vi "Configure Bus Monitor.vi"(6 "Starting Address Offset":u16 format="%04x", 7 "Virtual Memory Unit in":refnum<class "Virtual Memory Unit.lvclass">, 8 "error in (no error)":errorcluster, 11 "Bus Monitor in":refnum<class "Bus Monitor.lvclass">) -> (0 "error out":errorcluster, 3 "Bus Monitor out":refnum<class "Bus Monitor.lvclass">, 5 "Virtual Memory Unit out":refnum<class "Virtual Memory Unit.lvclass">)   [LabVIEW 2020, in "BCI-1553 API.lvlib" / "Bus Monitor.lvclass"]
doc: "Configures the Bus Monitor. The Bus Monitor defaults to every command being filtered out, with new commands being filtered in based on the filters contained in this Bus Monitor at this time. The Bus Monitor will make space for 250 commands (1000-2000 addresses) and 750 data fields (26250 addresses)."
uses:
  Bus Monitor.lvclass
  Dependencies/Virtual Memory Unit/Virtual Memory Unit.lvclass
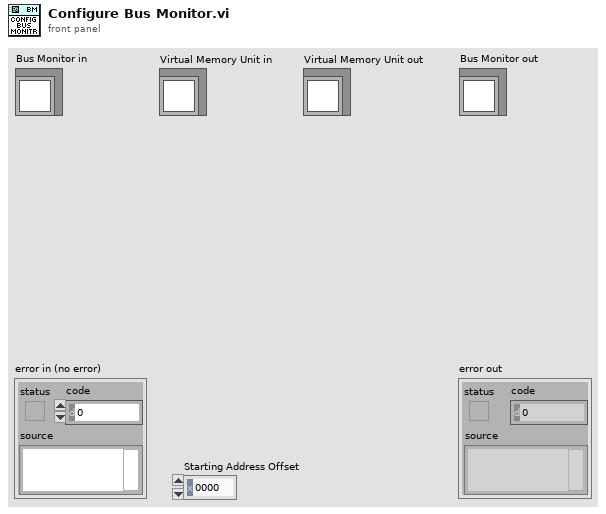
[diagram p1: front panel]
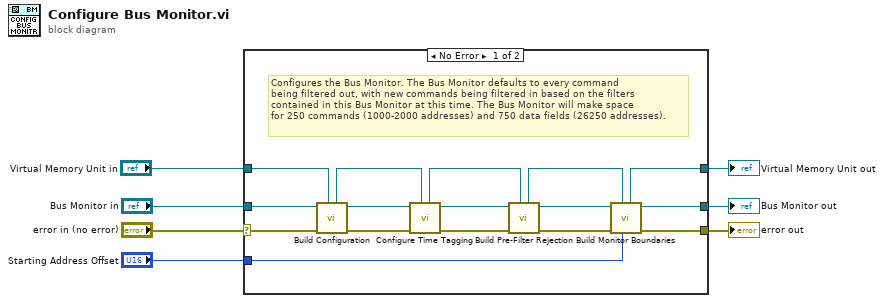
[diagram p0: block diagram]
diagram:
  n1 = case shown="No Error" "error in (no error)" {
    selector: "error in (no error)" -> [w21 w26]
    tunnel: [w17 w26] -> w6
    tunnel: [w15 w25] -> w4
    tunnel: "Bus Monitor in" -> [w20 w25]
    tunnel: "Virtual Memory Unit in" -> [w18 w24]
    tunnel: [w16 w24] -> w2
    tunnel: "Starting Address Offset" -> [w14 _]
    frame No Error {
      # "Configures the Bus Monitor. The Bus Monitor defaults to every command\nbeing filtered out, with new commands being filtered in based on the filters\ncontained in this Bus Monitor at this time. The Bus Monitor will make space\nfor 250 commands (1000-2000 addresses) and 750 data fields (26250 addresses)."
      n2 = call "Build Configuration.vi"("Virtual Memory Unit in"=w18, "error in (no error)"=w21, "Bus Monitor in"=w20) -> ("error out"=w11:errorcluster, "Bus Monitor out"=w13:refnum<class "Bus Monitor.lvclass">, "Virtual Memory Unit out"=w9:refnum<class "Virtual Memory Unit.lvclass">)  [unwired: 6 in]
      n3 = call "Configure Time Tagging.vi"("Virtual Memory Unit in"=w9, "error in (no error)"=w11, "Bus Monitor in"=w13) -> ("error out"=w10:errorcluster, "Bus Monitor out"=w12:refnum<class "Bus Monitor.lvclass">, "Virtual Memory Unit out"=w8:refnum<class "Virtual Memory Unit.lvclass">)  [unwired: 6 in]
      n4 = call "Build Pre-Filter Rejection.vi"("Virtual Memory Unit in"=w8, "error in (no error)"=w10, "Bus Monitor in"=w12) -> ("error out"=w22:errorcluster, "Bus Monitor out"=w23:refnum<class "Bus Monitor.lvclass">, "Virtual Memory Unit out"=w19:refnum<class "Virtual Memory Unit.lvclass">)  [unwired: 6 in]
      n5 = call "Build Monitor Boundaries.vi"("Starting Address Offset"=w14, "Virtual Memory Unit in"=w19, "error in (no error)"=w22, "Bus Monitor in"=w23) -> ("error out"=w17:errorcluster, "Bus Monitor out"=w15:refnum<class "Bus Monitor.lvclass">, "Virtual Memory Unit out"=w16:refnum<class "Virtual Memory Unit.lvclass">)  [unwired: 5 in]
    }
    frame Error {
    }
  }
  "error out" <- w6
  "Bus Monitor out" <- w4
  "Virtual Memory Unit out" <- w2
